vi "Sub_Init.vi"(8 "error in (no error)":errorcluster, 10 "String":string="Sub=%0.1f", 11 "Object in":refnum<class "Sub.lvclass">) -> (0 "error out":errorcluster, 3 "object out":refnum<class "Sub.lvclass">)   [LabVIEW 2019, in "Sub.lvclass"]
uses:
  Sub.lvclass
  C:/Program Files (x86)/National Instruments/LabVIEW 2019/examples/Open_GDS/GDS/InterfaceByViServer/Base_class/Base.lvclass
  Sub.lvclass/Sub.ctl
  Base_class/Base.lvclass
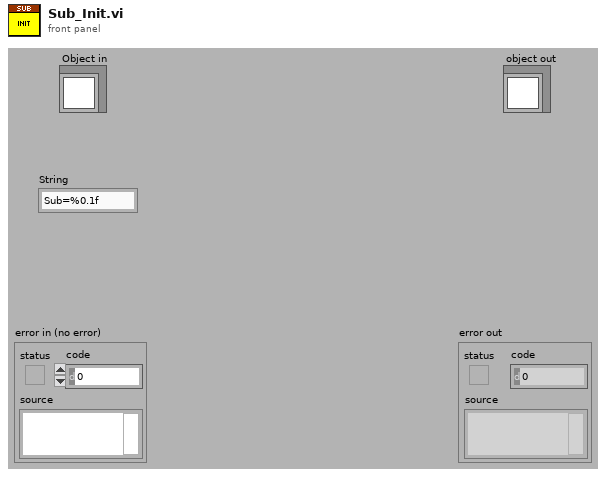
[diagram p1: front panel]
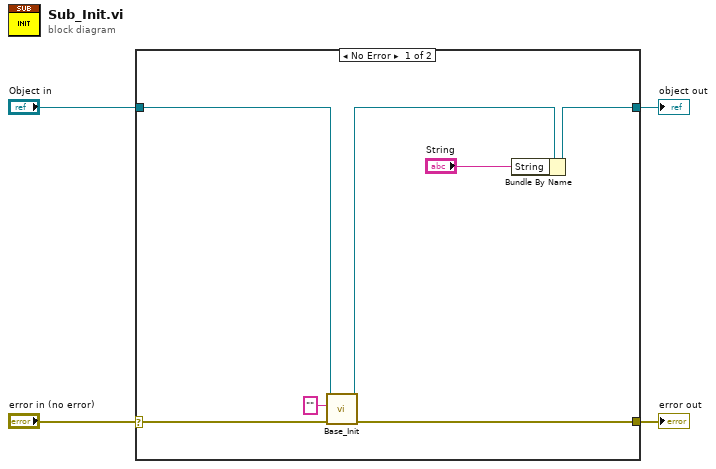
[diagram p0: block diagram]
diagram:
  n1 = case shown="No Error" "error in (no error)" {
    selector: "error in (no error)" -> [w10 w12]
    tunnel: [w11 w13] -> w4
    tunnel: "Object in" -> [w8 w13]
    tunnel: [w9 w12] -> w1
    frame No Error {
      n2 = call "Base_Init.vi"("error in (no error)"=w10, "String"="", "object in"=w8) -> ("error out"=w9:errorcluster, "object out"=w7:refnum<class "Sub.lvclass">)  [unwired: 7 in]
      n3 = Bundle By Name(cluster=w7, "String"="String") -> (w11:refnum<class "Sub.lvclass">)
    }
    frame Error {
    }
  }
  "object out" <- w4
  "error out" <- w1
